vi "Confirm Board Setup State.vi"(0 "Queue in":refnum<queue>, 9 "Test Results in":T2, 11 "error in (no error)":errorcluster) -> (4 "State":T1, 10 "Test Results out":T2, 15 "error out":errorcluster)   [LabVIEW 2016]
doc: "This VI promts the user as to wheteher or not the powers power supply and GEA2 connection are connected. If connected test proceeds to next state, if not test remains in this state until connected."
uses:
  C:/Program Files (x86)/National Instruments/LabVIEW 2016/examples/Design Patterns/Queued Message Handler/support/QMH Fundamentals - Message Cluster.ctl
  controls/Test Results.ctl
  controls/states.ctl
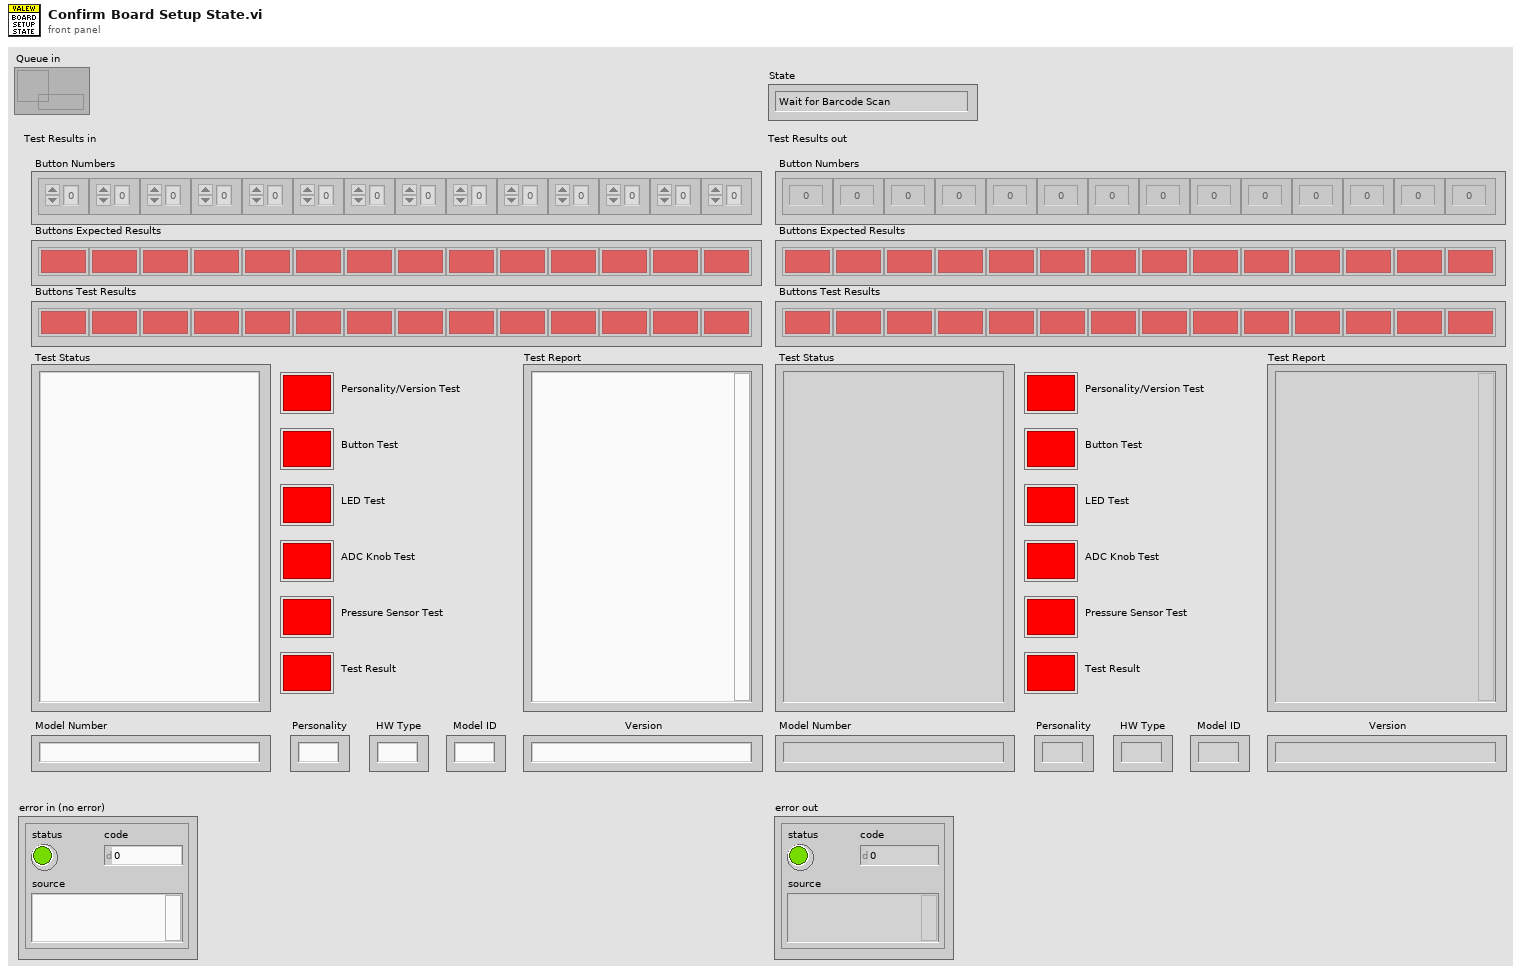
[diagram p1: front panel]
types:
  T1 = typedef "states.ctl" = enum16{"Wait for Barcode Scan", "Confirm Board Setup", "Initialization", "Perosnality Test", "Button Test", "LED Test", "ADC Knob Test", "Pressure Sensor Test", "Test Complete", "Log Results", "Re-Init Test", "Shutdown"}
  T2 = typedef "Test Results.ctl" = cluster{"Test Status":string, "Personality/Version Test ":bool, "Test Report":string, "Model Number":string, "Button Numbers":i32[], "Buttons Test Results":bool[], "Buttons Expected Results":bool[], "Model ID":string, "Personality":string, "HW Type":string, "Version":string, "Button Test":bool, "LED Test":bool, "ADC Knob Test":bool, "Pressure Sensor Test":bool, "Test Result":bool}
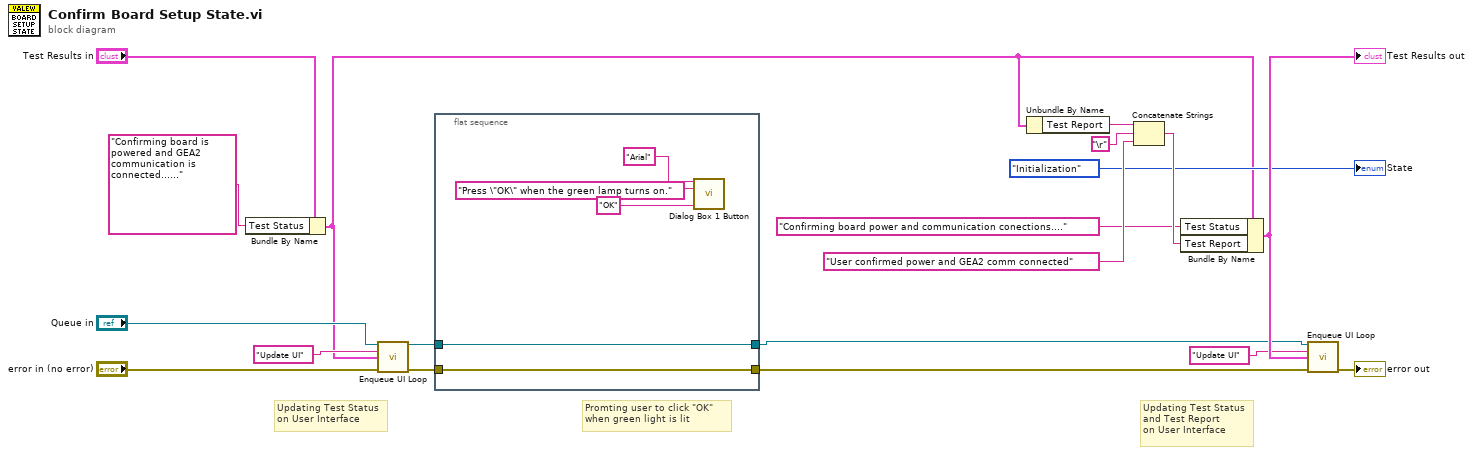
[diagram p0: block diagram]
diagram:
  # "Updating Test Status\nand Test Report\non User Interface"
  # "Promting user to click \"OK\"\nwhen green light is lit"
  # "Updating Test Status\non User Interface"
  n1 = Bundle By Name(cluster="Test Results in", "Test Status"="Confirming board is powered and GEA2 communication is connected......") -> (w6:T2)
  n2 = call "Enqueue UI Loop.vi"("UI Que In"="Queue in", "Message"="Update UI", "Test Results"=w6, "error in (no error)"="error in (no error)") -> ("UI Queue Out"=w3:refnum<queue>, "error out"=w2:errorcluster)  [unwired: 10 in]
  n3 = flat-sequence {
    tunnel: [w21] -> w4
    tunnel: w3 -> [w21]
    tunnel: w2 -> [w20]
    tunnel: [w20] -> w1
    frame #0 {
      n4 = call "Dialog Box 1 Button.vi"("Font Name"="Arial", "Input"="Press \"OK\" when the green lamp turns on.", "Button Name (\"OK\")"="OK" ("Button Name (\"OK\")")) -> ()  [unwired: 13 in]
    }
  }
  n5 = Unbundle By Name(w6) -> ("Test Report"=w13:string)
  n6 = Concatenate Strings(w13, "\r", "User confirmed power and GEA2 comm connected") -> (w16:string)
  n7 = Bundle By Name(cluster=w6, "Test Status"="Confirming board power and communication conections....", "Test Report"=w16) -> (w19:T2)
  "Test Results out" <- w19
  n8 = call "Enqueue UI Loop.vi"("UI Que In"=w4, "Message"="Update UI", "Test Results"=w19, "error in (no error)"=w1) -> ("error out"=→"error out":errorcluster)  [unwired: 10 in, 1 out]
  "State" <- states."Initialization" ("Enum")
